vi "splitcmd_func.vi"(0 "tasklist":string="r48[iR2000(z5.065,0.065m1d1800)_iG2000(z5.065,0.065m0d0)_iB2000(z5.065,0.065m0d0)_iP2000(z5.065,0.065m0d0)]\r\nr24[iR2000(z5.065,0.065m1d1800)_iG2000(z5.065,0.065m0d0)_iB2000(z5.065,0.065m0d0)_iP2000(z5.065,0.065m0d0)]\r\nr1[iR2000(z5.065,0.065m1d1800)_iG2000(z5.065,0.065m0d0)_iB2000(z5.065,0.065m0d0)_iP2000(z5.065,0.065m0d0)]\r\n", 5 "task ID":i32, 11 "error in":errorcluster) -> (3 "TaskNum":i32, 4 "R":cluster{i32, dbl, dbl, i32, i32}, 6 "G":cluster{i32, dbl, dbl, i32, i32}, 8 "B":cluster{i32, dbl, dbl, i32, i32}, 10 "P":cluster{i32, dbl, dbl, i32, i32}, 14 "r":i32, 15 "error out":errorcluster)   [LabVIEW 2024]
uses:
  <vilib>/Utility/error.llb/Trim Whitespace One-Sided.vi
panel:
  out "element":string
  out "cmd array":string[](array[string])
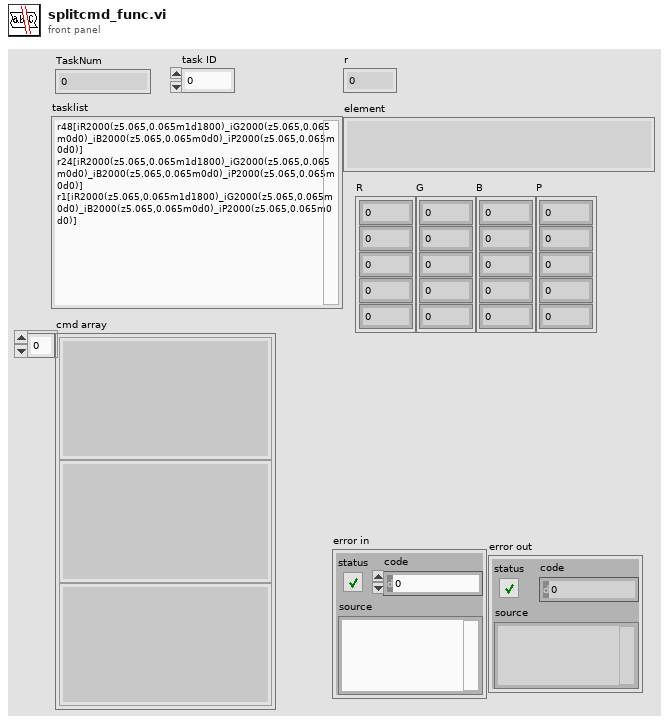
[diagram p1: front panel]
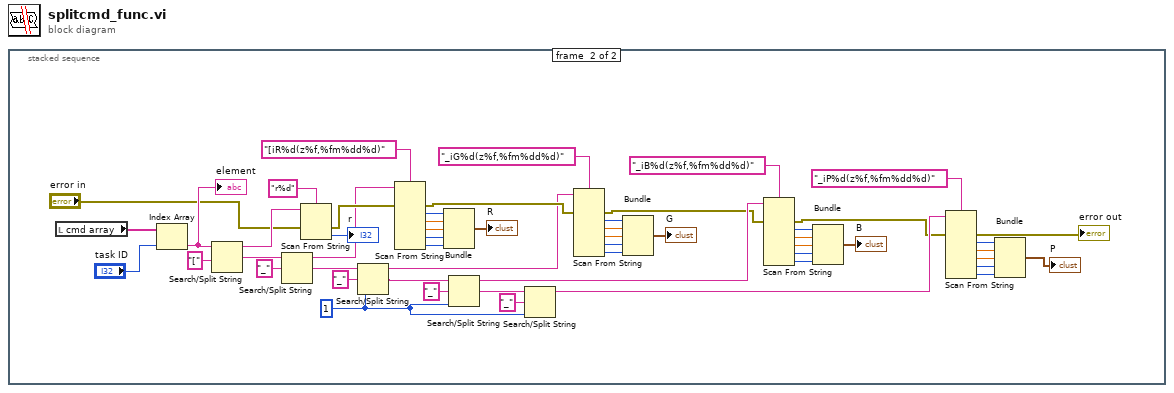
[diagram p0: block diagram]
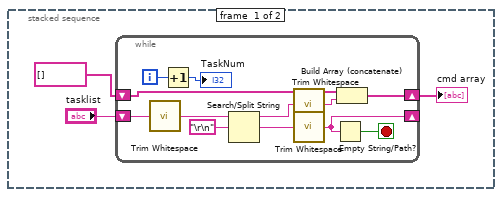
[diagram p2: hidden frame]
diagram:
  n1 = stacked-sequence {
    frame #0 {
      n2 = while {
        shift-right: [w10] -> _
        shift-left: "tasklist" -> [w15]
        shift-right: [w4] -> w1
        shift-left: string[] [] -> [w5]
        i -> [w12]
        stop <- w9 stop-if-true
        n3 = call <vilib>:"Trim Whitespace.vi"("string"=w15) -> ("trimmed string"=w14:string)  [unwired: 1 in]
        n4 = Increment(x=w12) -> (x+1=→"TaskNum":i32)
        n5 = Search/Split String(string=w14, search string/char (-)="\r\n") -> (substring before match=w7:string, match + rest of string=w11:string)  [unwired: 1 in, 1 out]
        n6 = call <vilib>:"Trim Whitespace.vi"("string"=w7) -> ("trimmed string"=w6:string)  [unwired: 1 in]
        n7 = call <vilib>:"Trim Whitespace.vi"("string"=w11) -> ("trimmed string"=w10:string)  [unwired: 1 in]
        n8 = Empty String/Path?(string/path=w10) -> (empty?=w9:bool)
        n9 = Build Array (concatenate)(w5, w6) -> (w4:string[])
      }
      "cmd array" <- w1
    }
    frame #1 {
      w17 = 1 ("offset (0)")
      n10 = local read "cmd array"() -> (w69:string[])
      n11 = Index Array(array=w69, index="task ID") -> (element=w67:string)
      "element" <- w67
      n12 = Search/Split String(string=w67, search string/char (-)="[") -> (substring before match=w64:string, match + rest of string=w66:string)  [unwired: 1 in, 1 out]
      n13 = Search/Split String(string=w66, search string/char (-)="_") -> (substring before match=w20:string, match + rest of string=w19:string)  [unwired: 1 in, 1 out]
      n14 = Scan From String(format string="r%d", input string=w64, error in="error in") -> (error out=w33:errorcluster, output 1=→"r":i32)  [unwired: 2 in, 2 out]
      n15 = Search/Split String(string=w19, search string/char (-)="_", offset (0)=w17) -> (substring before match=w18:string, match + rest of string=w57:string)  [unwired: 1 out]
      n16 = Scan From String(format string="[iR%d(z%f,%fm%dd%d)", input string=w20, error in=w33) -> (error out=w32:errorcluster, output 1=w55:i32, output 2=w54:dbl, output 3=w53:dbl, output 4=w52:i32, output 5=w51:i32)  [unwired: 6 in, 2 out]
      n17 = Bundle(w55, w54, w53, w52, w51) -> (→"R":cluster{i32, dbl, dbl, i32, i32})  [unwired: 1 in]
      n18 = Search/Split String(string=w57, search string/char (-)="_", offset (0)=w17) -> (substring before match=w35:string, match + rest of string=w59:string)  [unwired: 1 out]
      n19 = Search/Split String(string=w59, search string/char (-)="_", offset (0)=w17) -> (substring before match=w23:string)  [unwired: 2 out]
      n20 = Scan From String(format string="_iG%d(z%f,%fm%dd%d)", input string=w18, error in=w32) -> (error out=w31:errorcluster, output 1=w48:i32, output 2=w47:dbl, output 3=w46:dbl, output 4=w45:i32, output 5=w44:i32)  [unwired: 6 in, 2 out]
      n21 = Bundle(w48, w47, w46, w45, w44) -> (→"G":cluster{i32, dbl, dbl, i32, i32})  [unwired: 1 in]
      n22 = Scan From String(format string="_iB%d(z%f,%fm%dd%d)", input string=w35, error in=w31) -> (error out=w22:errorcluster, output 1=w41:i32, output 2=w40:dbl, output 3=w39:dbl, output 4=w38:i32, output 5=w37:i32)  [unwired: 6 in, 2 out]
      n23 = Bundle(w41, w40, w39, w38, w37) -> (→"B":cluster{i32, dbl, dbl, i32, i32})  [unwired: 1 in]
      n24 = Scan From String(format string="_iP%d(z%f,%fm%dd%d)", input string=w23, error in=w22) -> (error out=→"error out":errorcluster, output 1=w29:i32, output 2=w28:dbl, output 3=w27:dbl, output 4=w26:i32, output 5=w25:i32)  [unwired: 6 in, 2 out]
      n25 = Bundle(w29, w28, w27, w26, w25) -> (→"P":cluster{i32, dbl, dbl, i32, i32})  [unwired: 1 in]
    }
  }
